vi "List Open Front Panels__ogtk.vi"() -> (0 "Open Front Panels":string[](array[string]))   [LabVIEW 2012]
doc: "Returns an array of the names of all VIs in memory whose front panels are open."
panel:
  # "List Open Front Panels.vi\n\nReturns an array of the names of all VIs in memory whose front panels are open.\n\nPlease visit http://www.OpenG.org to learn about the\nOpen Source LabVIEW software movement.\n\nNOTICE -- YOU MUST LEAVE THIS NOTICE IN PLACE.  PER THE TERMS OF THE LICENSE BELOW, YOU MAY SUBLICENSE THIS SOFTWARE \nIN ANY WAY THAT DOES NOT CONFLICT WITH THIS LICENSE.\n\n### BSD License (http://www.opensource.org/licenses/bsd-license.php) Begin ###\n \nCopyright (c) 2002, Jim Kring <jim@jimkring.com>\n\nAll rights reserved.\n\nRedistribution and use in source and binary forms, with or without modification, are permitted provided that the following conditions are met:\n\n    * Redistributions of source code must retain the above copyright notice, this list of conditions and the following disclaimer.\n    * Redistributions in binary form must reproduce the above copyright notice, this list of conditions and the following disclaimer in the \n       documentation and/or other materials provided with the distribution.\n    * Neither the name of SciWare, James Kring, Inc., nor the names of its contributors may be used to endorse or promote products derived \n       from this software without specific prior written permission.\n\nTHIS SOFTWARE IS PROVIDED BY THE COPYRIGHT HOLDERS AND CONTRIBUTORS \"AS IS\" AND ANY EXPRESS OR IMPLIED WARRANTIES, \nINCLUDING, BUT NOT LIMITED TO, THE IMPLIED WARRANTIES OF MERCHANTABILITY AND FITNESS FOR A PARTICULAR PURPOSE ARE \nDISCLAIMED. IN NO EVENT SHALL THE COPYRIGHT OWNER OR CONTRIBUTORS BE LIABLE FOR ANY DIRECT, INDIRECT, INCIDENTAL,\n SPECIAL, EXEMPLARY, OR CONSEQUENTIAL DAMAGES (INCLUDING, BUT NOT LIMITED TO, PROCUREMENT OF SUBSTITUTE GOODS OR \nSERVICES; LOSS OF USE, DATA, OR PROFITS; OR BUSINESS INTERRUPTION) HOWEVER CAUSED AND ON ANY THEORY OF LIABILITY, \nWHETHER IN CONTRACT, STRICT LIABILITY, OR TORT (INCLUDING NEGLIGENCE OR OTHERWISE) ARISING IN ANY WAY OUT OF THE USE \nOF THIS SOFTWARE, EVEN IF ADVISED OF THE POSSIBILITY OF SUCH DAMAGE.\n\n### BSD License End ###"
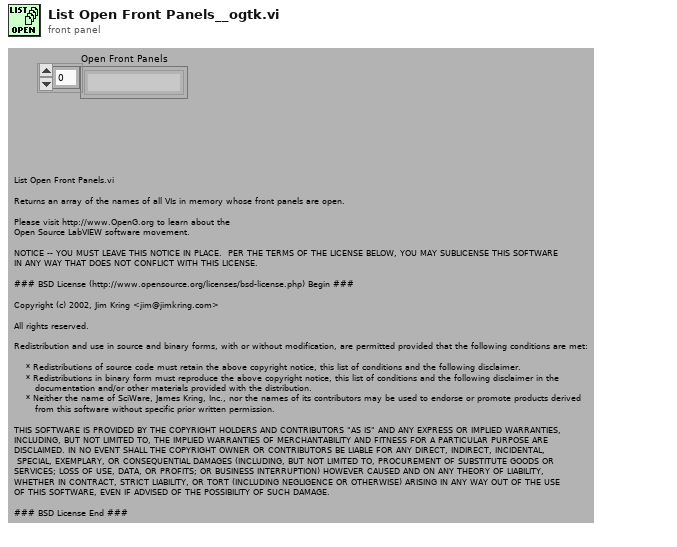
[diagram p1: front panel]
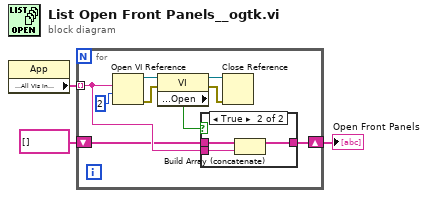
[diagram p0: block diagram]
diagram:
  n1 = property class="App"() -> ("Application:All VIs In Memory"=w3:string[])  [unwired: 2 in, 2 out]
  n2 = for {
    tunnel: w3 -> [w7] mode=indexing
    shift-right: [w5] -> w1
    shift-left: string[] [] ("Application:All VIs In Memory") -> [w6]
    n3 = Open VI Reference(vi path=w7, options=2) -> (vi reference=w12:refnum<vi>, error out=w11:errorcluster)  [unwired: 4 in]
    n4 = property class="VI"(reference=w12, error in=w11) -> (reference out=w10:refnum<vi>, error out=w9:errorcluster, "Front Panel Window:Open"=w8:bool)
    n5 = case shown="True" w8 {
      tunnel: w7 -> [_ w16]
      tunnel: w6 -> [w13 w15]
      tunnel: [w13 w14] -> w5
      frame False {
      }
      frame True {
        n6 = Build Array (concatenate)(w15, w16) -> (w14:string[])
      }
    }
    n7 = Close Reference(reference=w10, error in (no error)=w9) -> ()  [unwired: 1 out]
  }
  "Open Front Panels" <- w1
